vi "Newport ITX-D3N.vi"(8 "error in (no error)":errorcluster, 11 "Machine":string="192.168.1.161") -> (0 "error out":errorcluster, 3 "[Temp (F), RH]":dbl[](array[numeric]))   [LabVIEW 2011]
doc: "Demonstrates how to display an interactive send and receive message dialog for communication between TCP connections. It establishes a connection on the machine listed and the port specified. It then waits for you to input data into the Input Line string control and hit enter. Once you hit enter, the string you typed is sent to the port and passed to the TCP Communicator - Passive.vi where it is displayed on a string indicator.\n\nThe key difference between the Active and Passive VIs is that the Active VI establishes a connection, while the Passive VI waits for a connection to be established.\n\n<B>Note:</B> Requires the TCP Communicator - Passive.vi."
panel:
  out "Read Data":string
  out "Numeric":i32
  in  "Port":u16=2000
  # "Instructions:\n1. Open the TCP\n    Communicator - Passive.vi\n    and run it first.\n2. Run TCP Communicator - \n    Active.vi second.\n3.Type into the Input Line\n    String Control and then\n    hit Enter.\n4. Type into the Input Line\n    of the other VI and then\n    hit Enter.\n5. Press Stop to end session."
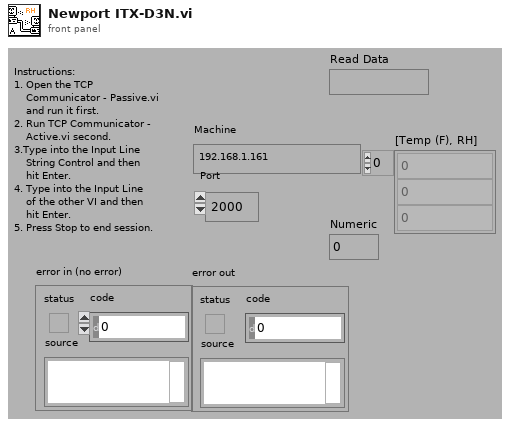
[diagram p1: front panel]
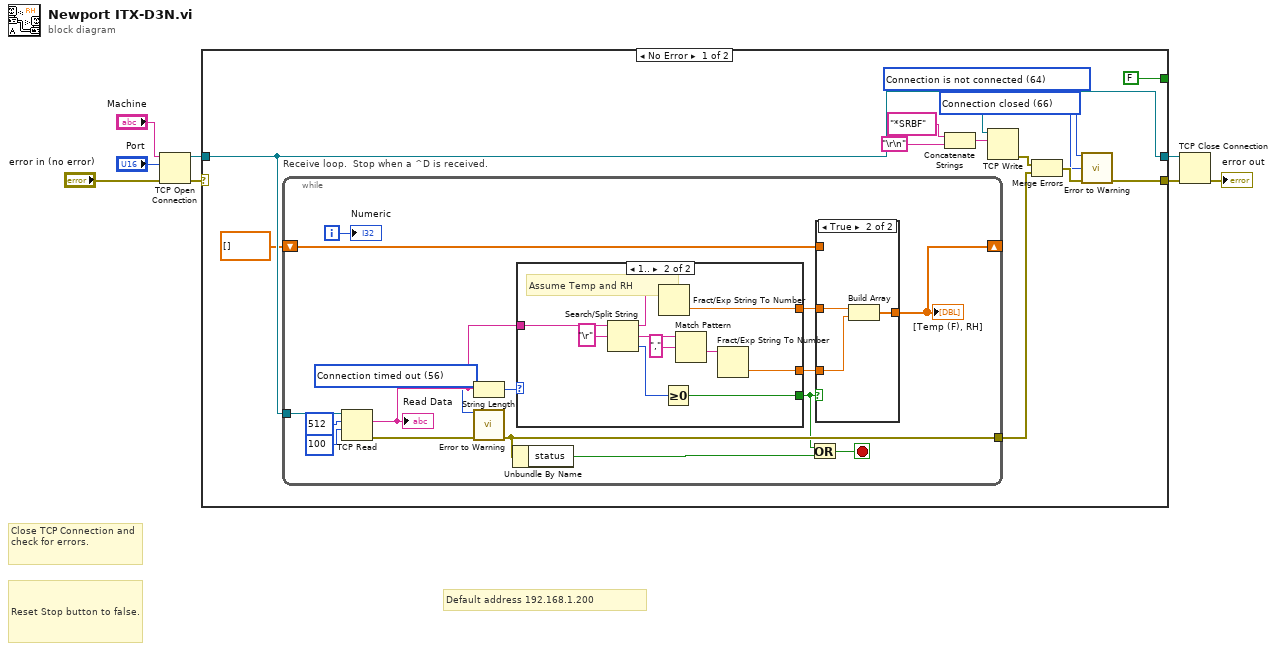
[diagram p0: block diagram]
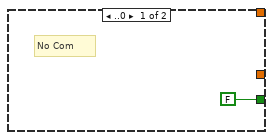
[diagram p3: hidden frame]
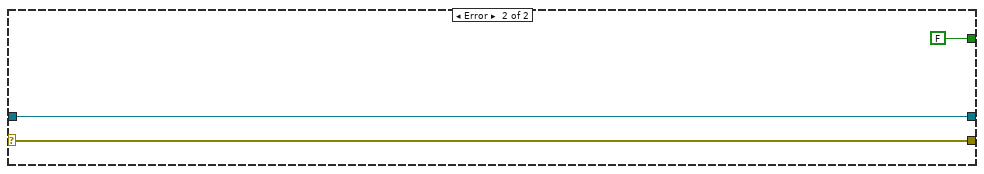
[diagram p4: hidden frame]
diagram:
  # "Default address 192.168.1.200"
  # "Close TCP Connection and check for errors."
  # "Reset Stop button to false."
  n1 = TCP Open Connection(address="Machine", remote port or service name="Port", error in (no error)="error in (no error)") -> (connection ID=w5:refnum<k5>, error out=w6:errorcluster)  [unwired: 2 in]
  n2 = case shown="No Error" w6 {
    selector: w6 -> [_ w53]
    tunnel: [w14 w53] -> w3
    tunnel: w5 -> [w20 w54]
    tunnel: [w20 w54] -> w4
    tunnel: [FALSE FALSE] -> _
    frame No Error {
      w15 = 66 items=["No Error", "Argument Error", "Memory Full", "Out of Zone", "End of File", "File Already Open", "Generic File IO Error", "File Not Found", "File Permission Error", "Disk Full", "Duplicate Path", "Too Many Files Open", "Not Enabled", "Resource File Not Found", "Cannot Add Resource", "Resource Not Found", "Image Not Found", "Image Memory Error", "Pen Does Not Exist", "Config Bad Type", "Config Token Not Found", "Config Parse Error", "Config Memory Error", "Bad External Code Format", "Bad External Code Offset", "External Code Not Present", "Null Window", "Destroy Window Mixup", "Null Menu", "Print Aborted", "Bad Print Record", "Print Driver Error", "Windows Error During Print", "Memory Error During Print", "Print Dialog Error", "Generic Print Error", "Invalid Device Refnum", "Device Not Found", "Device Parameter Error", "Device Unit Error", "Can't Open Device", "Device Call Aborted", "Generic Error", "Cancelled By User", "Object ID Too Low", "Object ID Too High", "Object Not In Heap", "Unknown Heap", "Bad DefProc ID", "DefProc Not In Table", "Message Out Of Range", "Null Method", "Unknown Message", "Manager Call Not Supported", "Bad address", "Connection In progress", "Connection timed out", "Connection is already in progress", "Network attribute not supported", "Network error", "Address in use", "System out of memory", "Connection aborted", "Connection refused", "Connection is not connected", "Connection is already connected", "Connection closed", "Initialize error (interapplication manager)", "Bad occurrence", "Wait on unbound occurrence handler", "Occurrence queue overflow", "Bad path", "Semaphore not signaled", "Unrecognized type (interapplication manager)"] ("3rd Error to Convert")
      w16 = 64 items=["No Error", "Argument Error", "Memory Full", "Out of Zone", "End of File", "File Already Open", "Generic File IO Error", "File Not Found", "File Permission Error", "Disk Full", "Duplicate Path", "Too Many Files Open", "Not Enabled", "Resource File Not Found", "Cannot Add Resource", "Resource Not Found", "Image Not Found", "Image Memory Error", "Pen Does Not Exist", "Config Bad Type", "Config Token Not Found", "Config Parse Error", "Config Memory Error", "Bad External Code Format", "Bad External Code Offset", "External Code Not Present", "Null Window", "Destroy Window Mixup", "Null Menu", "Print Aborted", "Bad Print Record", "Print Driver Error", "Windows Error During Print", "Memory Error During Print", "Print Dialog Error", "Generic Print Error", "Invalid Device Refnum", "Device Not Found", "Device Parameter Error", "Device Unit Error", "Can't Open Device", "Device Call Aborted", "Generic Error", "Cancelled By User", "Object ID Too Low", "Object ID Too High", "Object Not In Heap", "Unknown Heap", "Bad DefProc ID", "DefProc Not In Table", "Message Out Of Range", "Null Method", "Unknown Message", "Manager Call Not Supported", "Bad address", "Connection In progress", "Connection timed out", "Connection is already in progress", "Network attribute not supported", "Network error", "Address in use", "System out of memory", "Connection aborted", "Connection refused", "Connection is not connected", "Connection is already connected", "Connection closed", "Initialize error (interapplication manager)", "Bad occurrence", "Wait on unbound occurrence handler", "Occurrence queue overflow", "Bad path", "Semaphore not signaled", "Unrecognized type (interapplication manager)"] ("1st Error to Convert")
      n3 = while "Receive loop.  Stop when a ^D is received." {
        tunnel: [w29] -> w19
        tunnel: w20 -> [w34]
        shift-right: [w26] -> _
        shift-left: dbl[] [] -> [w22]
        i -> [w28]
        stop <- w25 stop-if-true
        w30 = 56 items=["No Error", "Argument Error", "Memory Full", "Out of Zone", "End of File", "File Already Open", "Generic File IO Error", "File Not Found", "File Permission Error", "Disk Full", "Duplicate Path", "Too Many Files Open", "Not Enabled", "Resource File Not Found", "Cannot Add Resource", "Resource Not Found", "Image Not Found", "Image Memory Error", "Pen Does Not Exist", "Config Bad Type", "Config Token Not Found", "Config Parse Error", "Config Memory Error", "Bad External Code Format", "Bad External Code Offset", "External Code Not Present", "Null Window", "Destroy Window Mixup", "Null Menu", "Print Aborted", "Bad Print Record", "Print Driver Error", "Windows Error During Print", "Memory Error During Print", "Print Dialog Error", "Generic Print Error", "Invalid Device Refnum", "Device Not Found", "Device Parameter Error", "Device Unit Error", "Can't Open Device", "Device Call Aborted", "Generic Error", "Cancelled By User", "Object ID Too Low", "Object ID Too High", "Object Not In Heap", "Unknown Heap", "Bad DefProc ID", "DefProc Not In Table", "Message Out Of Range", "Null Method", "Unknown Message", "Manager Call Not Supported", "Bad address", "Connection In progress", "Connection timed out", "Connection is already in progress", "Network attribute not supported", "Network error", "Address in use", "System out of memory", "Connection aborted", "Connection refused", "Connection is not connected", "Connection is already connected", "Connection closed", "Initialize error (interapplication manager)", "Bad occurrence", "Wait on unbound occurrence handler", "Occurrence queue overflow", "Bad path", "Semaphore not signaled", "Unrecognized type (interapplication manager)"] ("1st Error to Convert")
        n4 = TCP Read(connection ID=w34, bytes to read=512, 9:100) -> (data out=w33:string, error out=w31:errorcluster)  [unwired: 2 in, 1 out]
        "Read Data" <- w33
        n5 = String Length(string=w33) -> (length=w36:i32)
        n6 = call <vilib>:"Error to Warning.vi"("1st Error to Convert"=w30, "error in"=w31) -> ("warning out"=w29:errorcluster)  [unwired: 13 in]
        n7 = Unbundle By Name(w29) -> ("status"=w24:bool)
        n8 = case shown="1.." w36 {
          tunnel: w33 -> [_ w50]
          tunnel: [FALSE w49] -> w21
          tunnel: [_ w46] -> w27
          tunnel: [_ w45] -> w23
          frame ..0 {
            # "No Com"
          }
          frame 1.. {
            # "Assume Temp and RH"
            n9 = Search/Split String(string=w50, search string/char (-)="\r") -> (substring before match=w47:string, match + rest of string=w43:string, offset of match=w48:i32)  [unwired: 1 in]
            n10 = Fract/Exp String To Number(string=w47) -> (number=w46:dbl)  [unwired: 3 in, 1 out]
            n11 = Greater Or Equal To 0?(x=w48) -> (x >= 0?=w49:bool)
            n12 = Match Pattern(string=w43, regular expression="," ("search string/char (-)")) -> (after substring=w44:string)  [unwired: 1 in, 3 out]
            n13 = Fract/Exp String To Number(string=w44) -> (number=w45:dbl)  [unwired: 3 in, 1 out]
          }
        }
        n14 = Or(x=w21, y=w24) -> (x .or. y?=w25:bool)
        n15 = case shown="True" w21 {
          tunnel: w27 -> [_ w40]
          tunnel: [w37 w39] -> w26
          tunnel: w23 -> [_ w38]
          tunnel: w22 -> [w37 _]
          frame False {
          }
          frame True {
            n16 = Build Array(w40, w38) -> (w39:dbl[])
          }
        }
        "[Temp (F), RH]" <- w26
        "Numeric" <- w28
      }
      n17 = Concatenate Strings("*SRBF" ("Input Line"), "\r\n") -> (w10:string)
      n18 = TCP Write(connection ID=w20, data in=w10) -> (error out=w18:errorcluster)  [unwired: 2 in, 2 out]
      n19 = Merge Errors(w18, w19) -> (w17:errorcluster)
      n20 = call <vilib>:"Error to Warning.vi"("1st Error to Convert"=w16, "3rd Error to Convert"=w15, "error in"=w17) -> ("warning out"=w14:errorcluster)  [unwired: 12 in]
    }
    frame Error {
    }
  }
  n21 = TCP Close Connection(connection ID=w4, error in (no error)=w3) -> (error out=→"error out":errorcluster)  [unwired: 1 in, 1 out]
